vi "Configure Multi Eval Meas Power Dynamics Enabled.vi"(8 "error in (no error)":errorcluster, 9 "Enabled (Off)":bool, 10 "Instance (1)":T1=1, 11 "VISA resource name":refnum<visa-resource-name>) -> (0 "error out":errorcluster, 3 "VISA resource name out":refnum<visa-resource-name>)   [LabVIEW 2015, in "Rohde&Schwarz CMXP NR FR2 Measurement.lvlib"]
doc: "Enables or disables the evaluation of power dynamics results in the multi-evaluation measurement.\n\nAttribute:\nRSCMXPNRFR2M_ATTR_MULTI_EVAL_MEASUREMENT_POWER_DYNAMICS_ENABLED\n\nRemote-control command:\nCONFigure:NRMMw:MEAS<i>:MEValuation:RESult:PDYNamics"
uses:
  <instrlib>/Rohde&Schwarz CMXP NR FR2 Measurement/Rohde&Schwarz CMXP NR FR2 Measurement.lvlib
  <instrlib>/Rohde&Schwarz CMXP NR FR2 Measurement/Private/_Instance.ctl
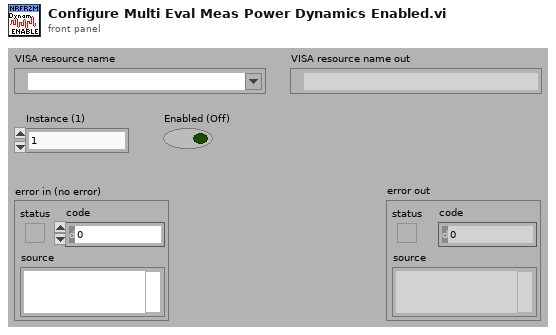
[diagram p1: front panel]
types:
  T1 = typedef "Rohde&Schwarz CMXP NR FR2 Measurement.lvlib/_Instance.ctl" = i32
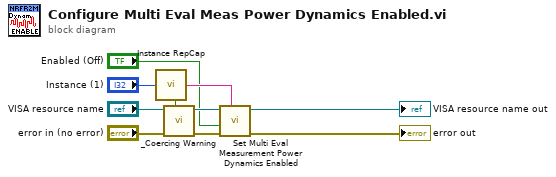
[diagram p0: block diagram]
diagram:
  n1 = call <instrlib>:"Instance RepCap.vi"("Instance In"="Instance (1)") -> ("In Range?"=w6:bool, "RepCap Identifier Out"=w5:string)  [unwired: 1 in]
  n2 = call <instrlib>:"_Coercing Warning.vi"("In Range?"=w6, "error in (no error)"="error in (no error)", "VISA resource name"="VISA resource name") -> ("error out"=w3:errorcluster, "VISA resource name out"=w4:refnum<visa-resource-name>)  [unwired: 7 in]
  n3 = call "Set Multi Eval Measurement Power Dynamics Enabled"("Repeated Capabilities"=w5, "error in (no error)"=w3, "Multi Eval Measurement Power Dynamics Enabled (OFF)"="Enabled (Off)", "instrument handle"=w4) -> ("error out"=→"error out":errorcluster, "instrument handle out"=→"VISA resource name out":refnum<visa-resource-name>)  [unwired: 6 in]
